vi "TLB Native Dynamic Events ver 0.04b alpha.vi"() -> ()   [LabVIEW 2018]
uses:
  Labview Training Phase 2/Enum Controls/States for Action Engine.ctl
  Type def/TLB event states.ctl
  Type def/TLB MHL States.ctl
panel:
  out "Action Queues":string[](array[string])
  out "State logic":T1
  out "Action State":string
  in  "Task condition":bool
  in  "Combo Box":string(combo)
  in  "Stop Queue":bool
  in  "Start Task":bool
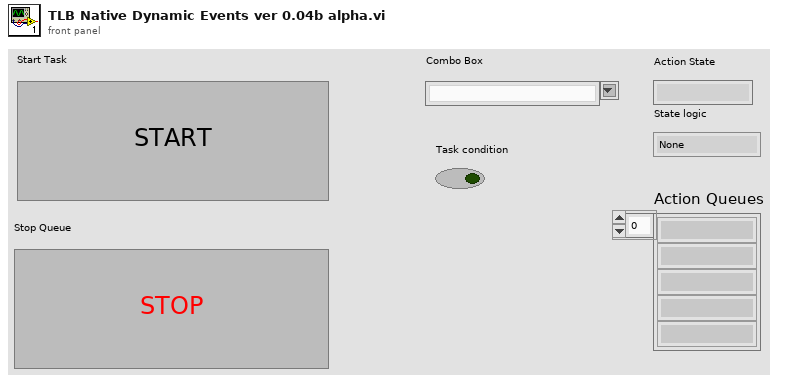
[diagram p1: front panel]
types:
  T1 = typedef "TLB MHL States.ctl" = enum16{"None", "Startup", "Idle", "Processing", "Shutdown", "Reset", "Task 1", "Task 2", "Task 3", "Task 4", "Task 4a", "Task 4b", "Task 4c", "Task 4d", "Task 4e", "Task 4f", "Task 4g", "Task 4h", "Acquire image", "Wall follow mode", "Autodrive", "Autodrive a"}
  T2 = typedef "States for Action Engine.ctl" = enum16{"Initialize", "Write", "Read"}
  T3 = typedef "TLB event states.ctl" = enum16{"Start Sequence", "Exit", "Start Task 1", "Start Task 2", "Start Task 3", "Start Task 4", "Camera vision", "Wall follow mode", "Idle", "Start Drive Straight"}
  T4 = typedef "TLB event states.ctl" = enum16{"Start Sequence", "Exit", "Task 1", "Task 2", "Idle"}
  T5 = cluster{"queue out":refnum<queue>, "error out":errorcluster}
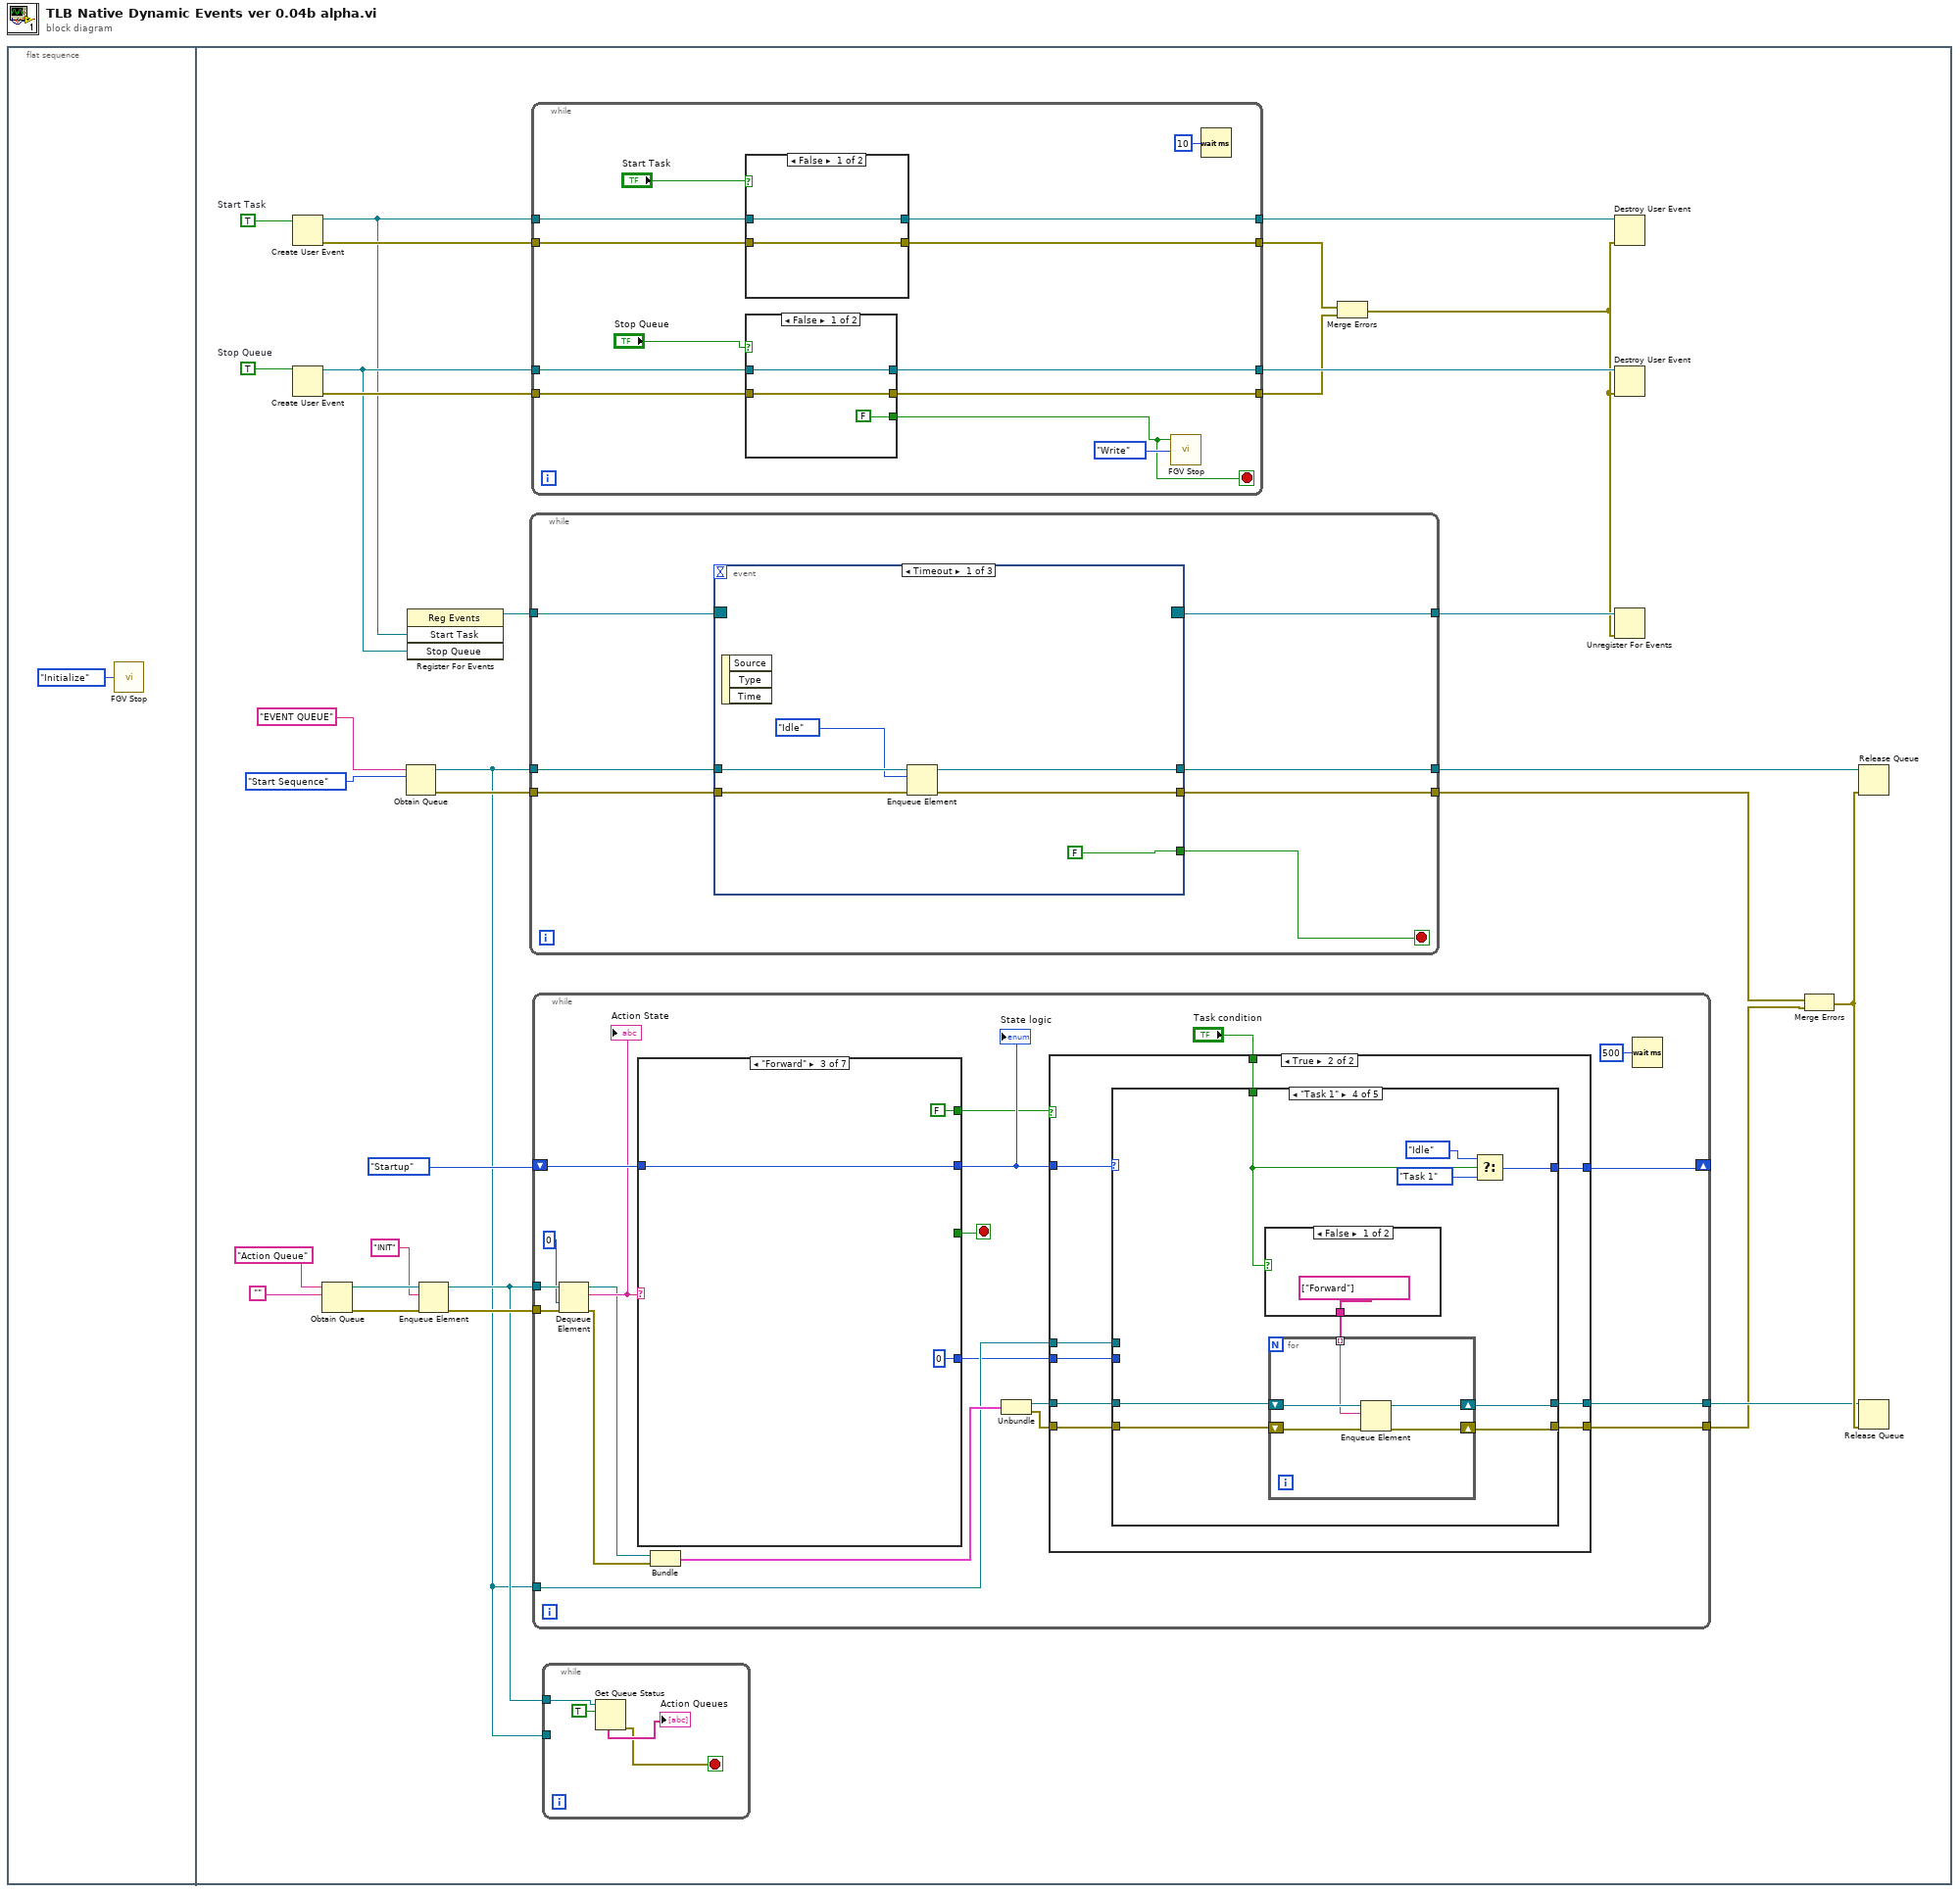
[diagram p0: block diagram]
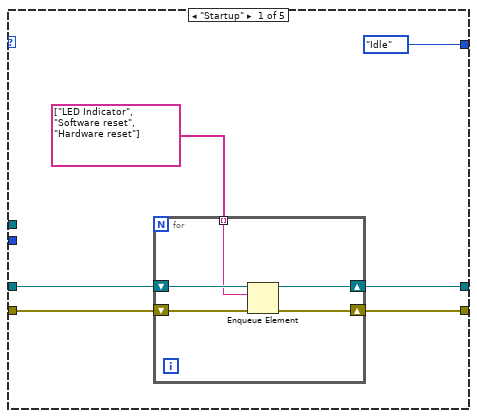
[diagram p3: hidden frame]
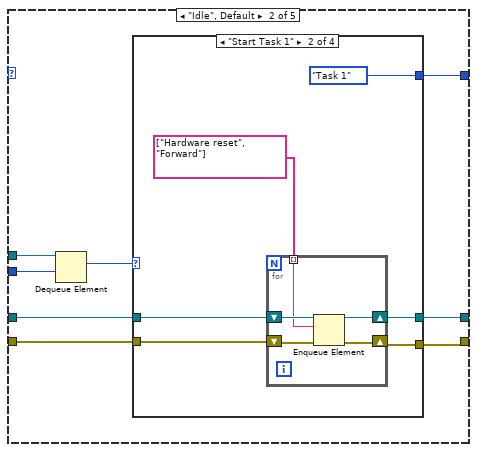
[diagram p4: hidden frame]
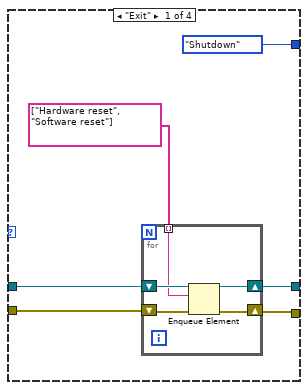
[diagram p5: hidden frame]
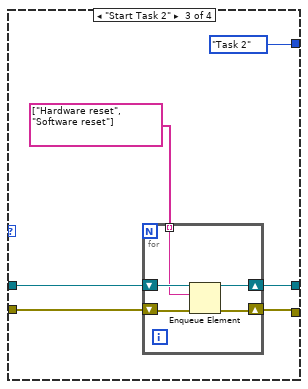
[diagram p6: hidden frame]
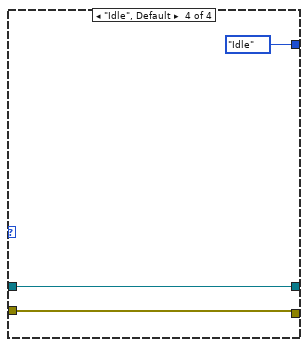
[diagram p7: hidden frame]
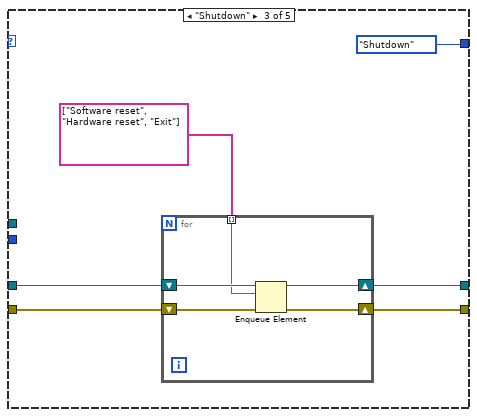
[diagram p8: hidden frame]
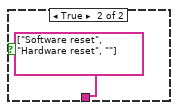
[diagram p9: hidden frame]
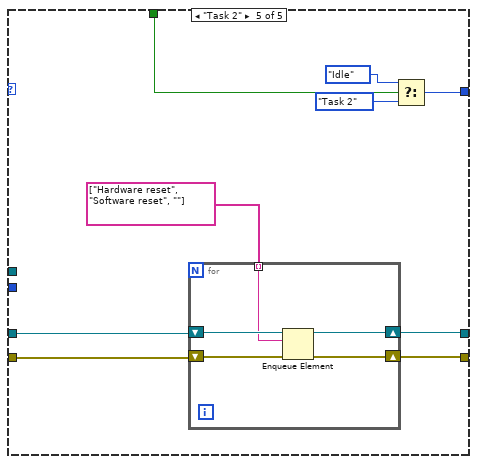
[diagram p10: hidden frame]
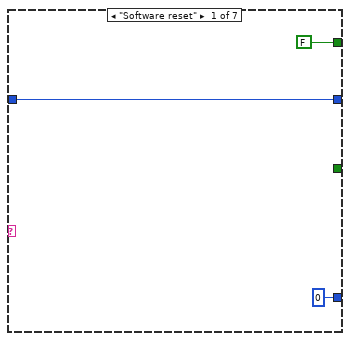
[diagram p11: hidden frame]
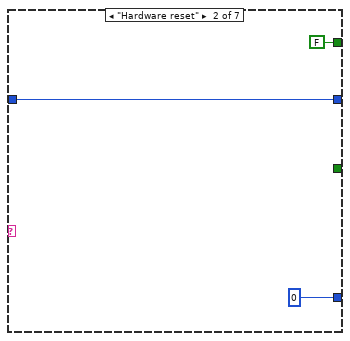
[diagram p12: hidden frame]
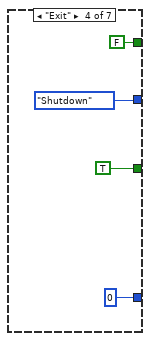
[diagram p13: hidden frame]
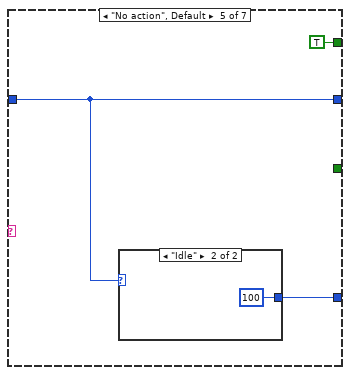
[diagram p14: hidden frame]
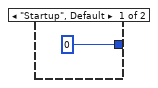
[diagram p15: hidden frame]
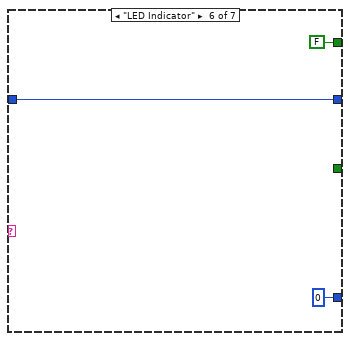
[diagram p16: hidden frame]
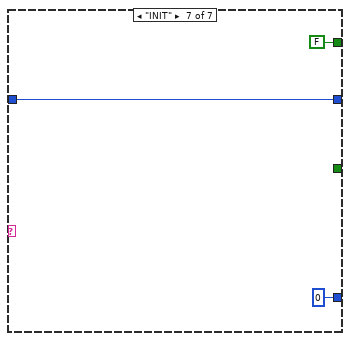
[diagram p17: hidden frame]
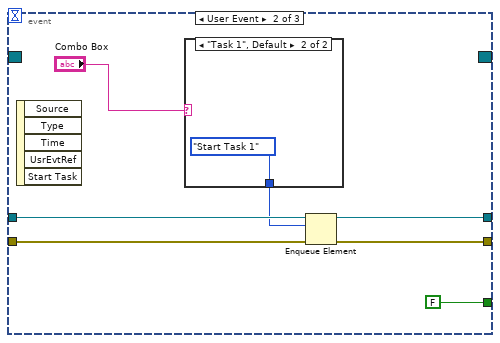
[diagram p18: hidden frame]
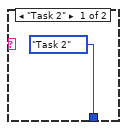
[diagram p19: hidden frame]
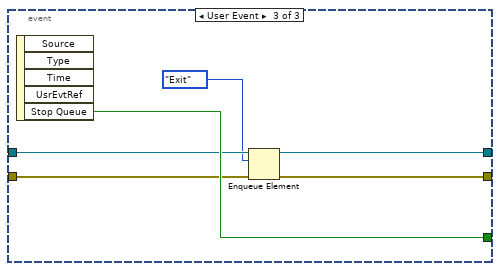
[diagram p20: hidden frame]
diagram:
  n1 = flat-sequence {
    frame #0 {
      n2 = call "FGV Stop.vi"("Init/Read/Write State"=States_for_Action_Engine."Initialize") -> ()  [unwired: 2 in, 2 out]
    }
    frame #1 {
      w31 = TRUE  # Stop Queue
      w30 = TRUE  # Start Task
      n3 = Create User Event(user event datatype=w30) -> (user event=w22:refnum<user-event>, error out=w27:errorcluster)  [unwired: 1 in]
      n4 = Create User Event(user event datatype=w31) -> (user event=w23:refnum<user-event>, error out=w26:errorcluster)  [unwired: 1 in]
      n5 = Obtain Queue(name (unnamed)="Action Queue", element data type="") -> (queue out=w15:refnum<queue>, error out=w11:errorcluster)  [unwired: 3 in, 1 out]
      n6 = Obtain Queue(name (unnamed)="EVENT QUEUE", element data type=TLB_event_states."Start Sequence" ("Enum")) -> (queue out=w2:refnum<queue>, error out=w12:errorcluster)  [unwired: 3 in, 1 out]
      n7 = register-events(w22, w23) -> (reference out=w21:refnum<event-registration>)  [unwired: 2 in, 1 out]
      n8 = Enqueue Element(queue=w15, element="INIT", error in (no error)=w11) -> (queue out=w3:refnum<queue>, error out=w10:errorcluster)  [unwired: 1 in, 1 out]
      n9 = while {
        tunnel: w21 -> [w194]
        tunnel: [w193] -> w20
        tunnel: w2 -> [w191]
        tunnel: [w190] -> w19
        tunnel: w12 -> [w189]
        tunnel: [w188] -> w9
        stop <- w192 stop-if-true
        n10 = event shown="[0] Timeout" {
          selector: w194 -> [_ _ _]
          dyn-events: [_ _ _] -> w193
          timeout: _ -> [_ _ _]
          tunnel: [FALSE FALSE w215] -> w192
          tunnel: w191 -> [w199 w206 w213]
          tunnel: [w198 w205 w214] -> w190
          tunnel: w189 -> [w196 w202 w211]
          tunnel: [w195 w201 w210] -> w188
          event Timeout {
            n11 = event-data() -> ()  [unwired: 1 in, 3 out]
            n12 = Enqueue Element(queue=w199, element=TLB_event_states."Idle" ("Enum"), error in (no error)=w196) -> (queue out=w198:refnum<queue>, error out=w195:errorcluster)  [unwired: 1 in, 1 out]
          }
          event User Event {
            n13 = event-data() -> ()  [unwired: 1 in, 5 out]
            n14 = case shown="\"Task 1\", Default" "Combo Box" {
              tunnel: [TLB_event_states."Task 2" ("Enum") TLB_event_states."Start Task 1" ("Enum")] -> w203
              frame "Task 2" {
              }
              frame "Task 1", Default {
              }
            }
            n15 = Enqueue Element(queue=w206, element=w203, error in (no error)=w202) -> (queue out=w205:refnum<queue>, error out=w201:errorcluster)  [unwired: 1 in, 1 out]
          }
          event User Event {
            n16 = event-data() -> ("Stop Queue"=w215:bool)  [unwired: 1 in, 4 out]
            n17 = Enqueue Element(queue=w213, element=TLB_event_states."Exit" ("Enum"), error in (no error)=w211) -> (queue out=w214:refnum<queue>, error out=w210:errorcluster)  [unwired: 1 in, 1 out]
          }
        }
      }
      n18 = while {
        tunnel: w22 -> [w227]
        tunnel: w23 -> [w226]
        tunnel: [w225] -> w29
        tunnel: [w224] -> w28
        tunnel: w27 -> [w223]
        tunnel: [w222] -> w25
        tunnel: w26 -> [w221]
        tunnel: [w220] -> w24
        stop <- w216 stop-if-true
        n19 = case shown="False" "Start Task" {
          selector: "Start Task" -> [_ w239]
          tunnel: w227 -> [w238 w243]
          tunnel: [w238 w242] -> w224
          tunnel: w223 -> [w237 w241]
          tunnel: [w237 w240] -> w222
          frame False {
          }
          frame True {
            n20 = Generate User Event(user event=w243, event data cluster=w239, error in=w241) -> (user event out=w242:refnum<user-event>, error out=w240:errorcluster)  [unwired: 1 in]
          }
        }
        n21 = case shown="False" "Stop Queue" {
          selector: "Stop Queue" -> [_ w232]
          tunnel: w226 -> [w231 w236]
          tunnel: [w231 w235] -> w225
          tunnel: w221 -> [w230 w234]
          tunnel: [w230 w233] -> w220
          tunnel: [FALSE w232] -> w216
          frame False {
          }
          frame True {
            n22 = Generate User Event(user event=w236, event data cluster=w232, error in=w234) -> (user event out=w235:refnum<user-event>, error out=w233:errorcluster)  [unwired: 1 in]
          }
        }
        n23 = call "FGV Stop.vi"("Init/Read/Write State"=States_for_Action_Engine."Write", "Input Node"=w216) -> ()  [unwired: 1 in, 2 out]
        n24 = Wait (ms)(milliseconds to wait=u32 10) -> ()  [unwired: 1 out]
      }
      n25 = while {
        tunnel: w2 -> [w41]
        shift-right: [w42] -> _
        shift-left: TLB_MHL_States."Startup" ("Enum") -> [w54]
        tunnel: w3 -> [w52]
        tunnel: w10 -> [w50]
        tunnel: [w44] -> w7
        tunnel: [w43] -> w6
        stop <- w39 stop-if-true
        n26 = Dequeue Element(queue=w52, timeout in ms (-1)=0, error in (no error)=w50) -> (queue out=w49:refnum<queue>, element=w51:string, error out=w48:errorcluster)  [unwired: 1 out]
        "Action State" <- w51
        n27 = case shown="\"Forward\"" w51 {
          tunnel: [w166 w169 w171 TLB_MHL_States."Shutdown" ("Enum") w179 w184 w187] -> w53
          tunnel: w54 -> [w166 w169 w171 _ w179 w184 w187]
          tunnel: [0 0 0 0 w178 0 0] -> w40
          tunnel: [_ _ _ TRUE _ _ _] -> w39
          tunnel: [FALSE FALSE FALSE FALSE TRUE FALSE FALSE] -> w37
          frame "Software reset" {
          }
          frame "Hardware reset" {
          }
          frame "Forward" {
          }
          frame "Exit" {
          }
          frame "No action", Default {
            n28 = case shown="\"Idle\"" w179 {
              tunnel: [0 100] -> w178
              frame "Startup", Default {
              }
              frame "Idle" {
              }
            }
          }
          frame "LED Indicator" {
          }
          frame "INIT" {
          }
        }
        "State logic" <- w53
        n29 = Bundle("queue out"=w49, "error out"=w48) -> (w47:T5)  [unwired: 1 in]
        n30 = Unbundle(w47) -> ("queue out"=w46:refnum<queue>, "error out"=w45:errorcluster)
        n31 = case shown="True" w37 {
          tunnel: w53 -> [w57 w67]
          tunnel: w46 -> [w58 w66]
          tunnel: w45 -> [w56 w65]
          tunnel: [w58 w64] -> w44
          tunnel: [w56 w63] -> w43
          tunnel: [w57 w62] -> w42
          tunnel: w41 -> [_ w61]
          tunnel: w40 -> [_ w60]
          tunnel: "Task condition" -> [_ w59]
          frame False {
          }
          frame True {
            n32 = case shown="\"Task 1\"" w67 {
              tunnel: w66 -> [w73 w80 w126 w137 w152]
              tunnel: w65 -> [w72 w82 w124 w136 w151]
              tunnel: [w71 w83 w125 w139 w154] -> w64
              tunnel: [w70 w81 w123 w138 w153] -> w63
              tunnel: [TLB_MHL_States."Idle" ("Enum") w84 TLB_MHL_States."Shutdown" ("Enum") w140 w156] -> w62
              tunnel: w61 -> [_ w86 _ _ _]
              tunnel: w60 -> [_ w79 _ _ _]
              tunnel: w59 -> [_ _ _ w135 w150]
              frame "Startup" {
                n33 = for {
                  shift-right: [w76] -> w71
                  shift-left: w73 -> [w78]
                  shift-right: [w75] -> w70
                  shift-left: w72 -> [w77]
                  tunnel: string[] ["LED Indicator", "Software reset", "Hardware reset"] -> [w74] mode=indexing
                  n34 = Enqueue Element(queue=w78, element=w74, error in (no error)=w77) -> (queue out=w76:refnum<queue>, error out=w75:errorcluster)  [unwired: 1 in, 1 out]
                }
              }
              frame "Idle", Default {
                n35 = Dequeue Element(queue=w86, timeout in ms (-1)=w79) -> (element=w85:T3)  [unwired: 1 in, 3 out]
                n36 = case shown="\"Start Task 1\"" w85 {
                  tunnel: [TLB_MHL_States."Shutdown" ("Enum") TLB_MHL_States."Task 1" ("Enum") TLB_MHL_States."Task 2" ("Enum") TLB_MHL_States."Idle" ("Enum")] -> w84
                  tunnel: [w89 w102 w111 w121] -> w83
                  tunnel: w80 -> [w91 w101 w113 w121]
                  tunnel: w82 -> [w90 w100 w112 w120]
                  tunnel: [w88 w99 w110 w120] -> w81
                  frame "Exit" {
                    n37 = for {
                      shift-right: [w97] -> w89
                      shift-left: w91 -> [w96]
                      shift-right: [w94] -> w88
                      shift-left: w90 -> [w95]
                      tunnel: string[] ["Hardware reset", "Software reset"] -> [w93] mode=indexing
                      n38 = Enqueue Element(queue=w96, element=w93, error in (no error)=w95) -> (queue out=w97:refnum<queue>, error out=w94:errorcluster)  [unwired: 1 in, 1 out]
                    }
                  }
                  frame "Start Task 1" {
                    n39 = for {
                      shift-right: [w108] -> w102
                      shift-left: w101 -> [w107]
                      shift-right: [w105] -> w99
                      shift-left: w100 -> [w106]
                      tunnel: string[] ["Hardware reset", "Forward"] -> [w104] mode=indexing
                      n40 = Enqueue Element(queue=w107, element=w104, error in (no error)=w106) -> (queue out=w108:refnum<queue>, error out=w105:errorcluster)  [unwired: 1 in, 1 out]
                    }
                  }
                  frame "Start Task 2" {
                    n41 = for {
                      shift-right: [w119] -> w111
                      shift-left: w113 -> [w118]
                      shift-right: [w116] -> w110
                      shift-left: w112 -> [w117]
                      tunnel: string[] ["Hardware reset", "Software reset"] -> [w115] mode=indexing
                      n42 = Enqueue Element(queue=w118, element=w115, error in (no error)=w117) -> (queue out=w119:refnum<queue>, error out=w116:errorcluster)  [unwired: 1 in, 1 out]
                    }
                  }
                  frame "Idle", Default {
                  }
                }
              }
              frame "Shutdown" {
                n43 = for {
                  shift-right: [w131] -> w125
                  shift-left: w126 -> [w133]
                  shift-right: [w130] -> w123
                  shift-left: w124 -> [w132]
                  tunnel: string[] ["Software reset", "Hardware reset", "Exit"] -> [w129] mode=indexing
                  n44 = Enqueue Element(queue=w133, element=w129, error in (no error)=w132) -> (queue out=w131:refnum<queue>, error out=w130:errorcluster)  [unwired: 1 in, 1 out]
                }
              }
              frame "Task 1" {
                n45 = case shown="False" w135 {
                  tunnel: [string[] ["Forward"] string[] ["Software reset", "Hardware reset", ""]] -> w134
                  frame False {
                  }
                  frame True {
                  }
                }
                n46 = for {
                  shift-right: [w147] -> w139
                  shift-left: w137 -> [w149]
                  shift-right: [w146] -> w138
                  shift-left: w136 -> [w148]
                  tunnel: w134 -> [w145] mode=indexing
                  n47 = Enqueue Element(queue=w149, element=w145, error in (no error)=w148) -> (queue out=w147:refnum<queue>, error out=w146:errorcluster)  [unwired: 1 in, 1 out]
                }
                n48 = Select(t=TLB_MHL_States."Idle" ("Enum"), s=w135, f=TLB_MHL_States."Task 1" ("Enum")) -> (s? t:f=w140:T1)
              }
              frame "Task 2" {
                n49 = for {
                  shift-right: [w161] -> w154
                  shift-left: w152 -> [w163]
                  shift-right: [w160] -> w153
                  shift-left: w151 -> [w162]
                  tunnel: string[] ["Hardware reset", "Software reset", ""] -> [w159] mode=indexing
                  n50 = Enqueue Element(queue=w163, element=w159, error in (no error)=w162) -> (queue out=w161:refnum<queue>, error out=w160:errorcluster)  [unwired: 1 in, 1 out]
                }
                n51 = Select(t=TLB_MHL_States."Idle" ("Enum"), s=w150, f=TLB_MHL_States."Task 2" ("Enum")) -> (s? t:f=w156:T1)
              }
            }
          }
        }
        n52 = Wait (ms)(milliseconds to wait=u32 500) -> ()  [unwired: 1 out]
      }
      n53 = while {
        tunnel: w3 -> [w33]
        tunnel: w2 -> [_]
        stop <- w32 stop-if-true
        n54 = Get Queue Status(queue=w33, return elements? (F)=TRUE) -> (error out=w32:errorcluster, elements=→"Action Queues":string[])  [unwired: 1 in, 6 out]
      }
      n55 = Merge Errors(w25, w24) -> (w5:errorcluster)
      n56 = Destroy User Event(user event=w28, error in=w5) -> ()  [unwired: 1 out]
      n57 = Destroy User Event(user event=w29, error in=w5) -> ()  [unwired: 1 out]
      n58 = Unregister For Events(event registration refnum=w20, error in=w5) -> ()  [unwired: 1 out]
      n59 = Merge Errors(w9, w6) -> (w8:errorcluster)
      n60 = Release Queue(queue=w19, error in (no error)=w8) -> ()  [unwired: 1 in, 3 out]
      n61 = Release Queue(queue=w7, error in (no error)=w8) -> ()  [unwired: 1 in, 3 out]
    }
  }
